vi "LOER_AdaptToInputs.vi"(0 "XRef":T9, 1 "Term Types":T6, 2 "State In":T1={"Inputs"=1, "SelectedIndex"=0, "ClassInfo"=[], "Width"=100, "EventReg Type"=variant}) -> (14 "Reply":T4, 15 "Fatal Error Out":T3, 16 "State Out":T1={"Inputs"=1, "SelectedIndex"=0, "ClassInfo"=[], "Width"=100, "EventReg Type"=variant})   [LabVIEW 2016, in "LV Object Event Registration Node.xnode"]
uses:
  LV Object Event Registration Node.xnode
  <vilib>/XNodeSupport/XNodeXNodeRef.ctl
  <vilib>/XNodeSupport/XNodeTermTypeIDPairs.ctl
  <vilib>/XNodeSupport/XNodeTermTypeIDPair.ctl
  <vilib>/XNodeSupport/XNodeType.ctl
  <vilib>/XNodeSupport/XNodeString.ctl
  LOER_State.ctl
  LOER_ClassInfo.ctl
  <vilib>/XNodeSupport/XNodeStringArray.ctl
  <vilib>/XNodeSupport/XNodeErrorCluster.ctl
  <vilib>/Utility/Data Type/NI_Data Type.lvlib
  <vilib>/XNodeSupport/NI_XNodeSupport.lvlib
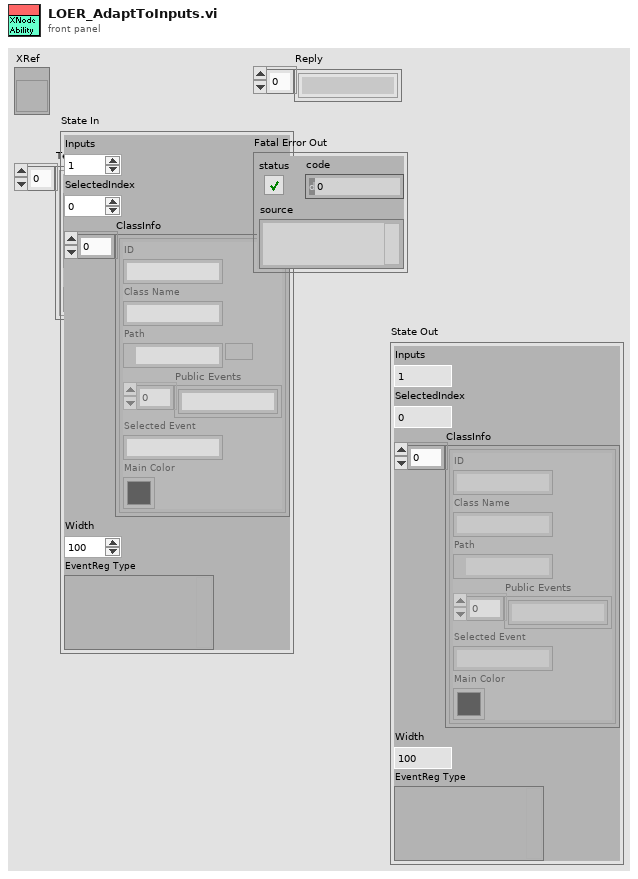
[diagram p1: front panel]
types:
  T1 = typedef "LV Object Event Registration Node.xnode/LOER_State.ctl" = cluster{"Inputs":u16, "SelectedIndex":i16, "ClassInfo":T2[], "Width":u16, "EventReg Type":variant}
  T2 = typedef "LV Object Event Registration Node.xnode/LOER_ClassInfo.ctl" = cluster{"ID":string, "Class Name":string, "Path":path, "Public Events":string[], "Selected Event":string, "Main Color":u32}
  T3 = typedef "NI_XNodeSupport.lvlib/XNodeErrorCluster.ctl" = errorcluster
  T4 = typedef "NI_XNodeSupport.lvlib/XNodeStringArray.ctl" = T5[]
  T5 = typedef "NI_XNodeSupport.lvlib/XNodeString.ctl" = string
  T6 = typedef "NI_XNodeSupport.lvlib/XNodeTermTypeIDPairs.ctl" = T7[]
  T7 = typedef "NI_XNodeSupport.lvlib/XNodeTermTypeIDPair.ctl" = cluster{"Type":T8, "Id":T5}
  T8 = typedef "NI_XNodeSupport.lvlib/XNodeType.ctl" = variant
  T9 = typedef "NI_XNodeSupport.lvlib/XNodeXNodeRef.ctl" = refnum<vi>
  T10 = typedef "LV Object Event Registration Node.xnode/LOERN_ClassInfo.ctl" = cluster{"ID":string, "Class Name":string, "Path":path, "Public Events":string[], "Selected Event":string, "Main Color":u32}
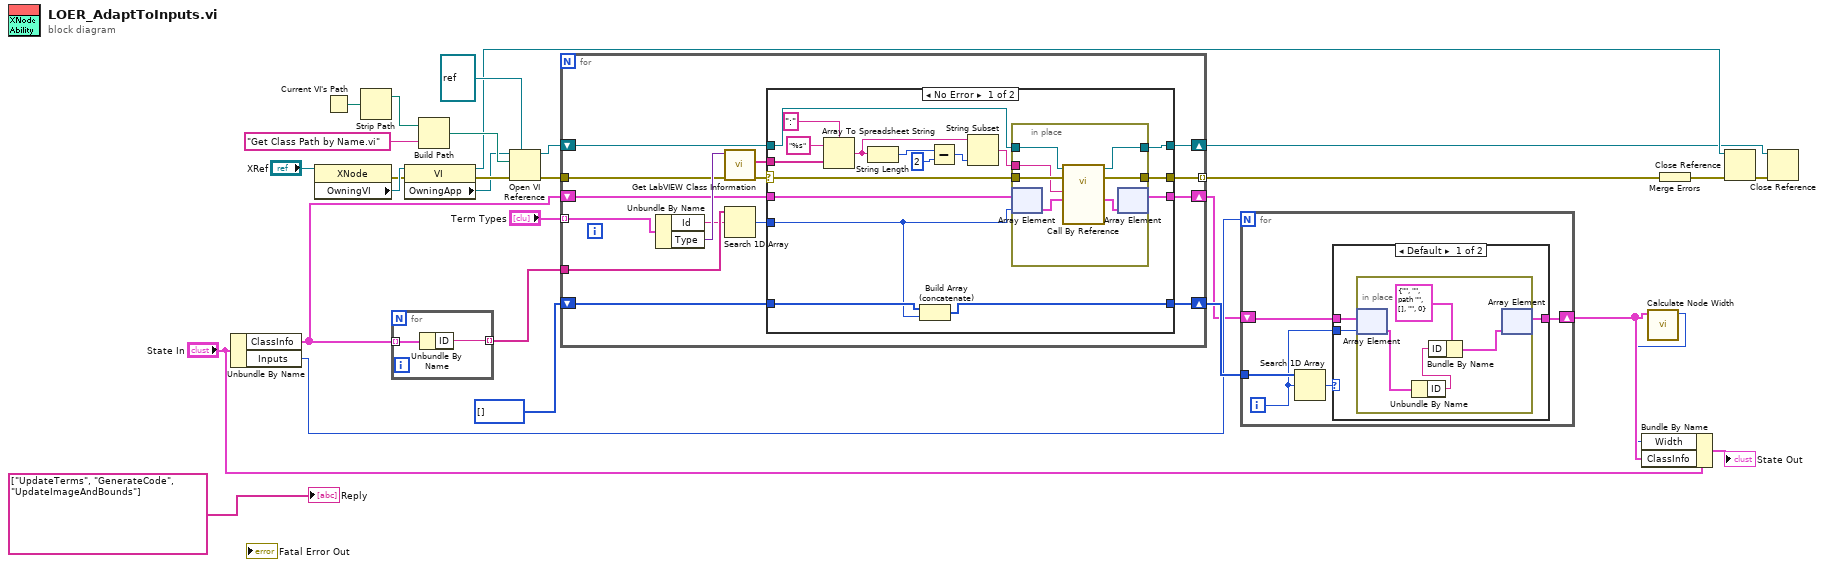
[diagram p0: block diagram]
diagram:
  n1 = Unbundle By Name("State In") -> ("ClassInfo"=w28:T2[], "Inputs"=w4:u16)
  n2 = property class="XNode"(reference="XRef") -> (error out=w22:errorcluster, "OwningVI"=w26:refnum<vi>)  [unwired: 1 in, 1 out]
  n3 = Current VI's Path() -> (path=w21:path)
  n4 = Strip Path(path=w21) -> (stripped path=w20:path)  [unwired: 1 out]
  n5 = for {
    tunnel: w28 -> [w31] mode=indexing
    tunnel: [w30] -> w29 mode=indexing
    n6 = Unbundle By Name(w31) -> ("ID"=w30:string)
  }
  n7 = property class="VI"(reference=w26, error in=w22) -> (reference out=w13:refnum<vi>, error out=w23:errorcluster, "OwningApp"=w17:refnum<vi>)
  n8 = Build Path(base path=w20, name or relative path="Get Class Path by Name.vi") -> (appended path=w18:path)
  n9 = Open VI Reference(type specifier VI Refnum (for type only)=refnum<vi> refnum, application reference (local)=w17, vi path=w18, error in (no error)=w23) -> (vi reference=w10:refnum<vi>, error out=w24:errorcluster)  [unwired: 2 in]
  n10 = for {
    tunnel: "Term Types" -> [w32] mode=indexing
    tunnel: w29 -> [w46]
    shift-right: [w35] -> w3
    shift-left: w28 -> [w36]
    tunnel: w24 -> [w43]
    shift-right: [w37] -> w8
    shift-left: w10 -> [w40]
    tunnel: [w38] -> w15 mode=indexing
    shift-right: [w33] -> w5
    shift-left: i32[] [] -> [w34]
    n11 = Unbundle By Name(w32) -> ("Id"=w42:T5, "Type"=w45:T8)
    n12 = call <vilib>:"Get LabVIEW Class Information.vi"("error in (no error)"=w43, "Variant"=w45) -> ("error out"=w39:errorcluster, "Qualified LabVIEW Class Name"=w44:string[])  [unwired: 7 in, 1 out]
    n13 = Search 1D Array(1D array=w46, element=w42) -> (index of element=w41:i32)  [unwired: 1 in]
    n14 = case shown="No Error" w39 {
      selector: w39 -> [w55 _]
      tunnel: w44 -> [w61 _]
      tunnel: w41 -> [w48 _]
      tunnel: w40 -> [w56 w73]
      tunnel: [w54 _] -> w38
      tunnel: [w53 w73] -> w37
      tunnel: w36 -> [w52 w71]
      tunnel: [w50 w71] -> w35
      tunnel: w34 -> [w49 w72]
      tunnel: [w47 w72] -> w33
      frame No Error {
        n15 = Array To Spreadsheet String(delimiter (Tab)=":", array=w61, 3:"%s" ("format string")) -> (spreadsheet string=w60:string)
        n16 = String Length(string=w60) -> (length=w59:i32)
        n17 = Build Array (concatenate)(w49, w48) -> (w47:i32[])
        n18 = Subtract(x=w59, y=2) -> (x-y=w57:i32)
        n19 = String Subset(string=w60, length (rest)=w57) -> (substring=w51:string)  [unwired: 1 in]
        n20 = in-place {
          in-place-border: w56 -> [w70]
          in-place-border: w55 -> [w69]
          in-place-border: [w68] -> w54
          in-place-border: [w67] -> w53
          in-place-border: w51 -> [w64]
          n21 = in-place-array #1(w52, w48) -> (w65:T2)
          n22 = call-by-ref "?"(reference=w70, error in=w69, "Original ClassInfo"=w65, "String"=w64) -> (reference out=w67:refnum<vi>, error out=w68:errorcluster, "output cluster"=w66:T10)  [unwired: 8 in, 1 out]
          n23 = in-place-array #1(w66) -> (w50:T2[])  [unwired: 1 out]
        }
      }
      frame Error {
      }
    }
  }
  n24 = for {
    N: w4 -> [_]
    tunnel: w5 -> [w78]
    shift-right: [w76] -> w2
    shift-left: w3 -> [w77]
    i -> [w74]
    n25 = Search 1D Array(1D array=w78, element=w74) -> (index of element=w75:i32)  [unwired: 1 in]
    n26 = case shown="Default" w75 {
      tunnel: w77 -> [w81 w86]
      tunnel: [w79 w86] -> w76
      tunnel: w74 -> [w80 _]
      frame Default {
        n27 = in-place {
          n28 = in-place-array #2(w81, w80) -> (w84:T2)
          n29 = Unbundle By Name(w84) -> ("ID"=w82:string)
          n30 = Bundle By Name(cluster=T2 {"ID"="", "Class Name"="", "Path"=path "", "Public Events"=[], "Selected Event"="", "Main Color"=0} ("new element/subarray"), "ID"=w82) -> (w85:T2)
          n31 = in-place-array #2(w85) -> (w79:T2[])  [unwired: 1 out]
        }
      }
      frame 0.. {
      }
    }
  }
  n32 = call "Calculate Node Width.vi"("ClassInfo"=w2) -> ("upper limit"=w1:i16)  [unwired: 10 in]
  n33 = Bundle By Name(cluster="State In", "Width"=w1, "ClassInfo"=w2) -> (→"State Out":T1)
  n34 = Merge Errors(w15) -> (w14:errorcluster)
  n35 = Close Reference(reference=w13, error in (no error)=w14) -> (error out=w9:errorcluster)
  n36 = Close Reference(reference=w8, error in (no error)=w9) -> ()  [unwired: 1 out]
  "Reply" <- T4 ["UpdateTerms", "GenerateCode", "UpdateImageAndBounds"] ("Reply")
